vi "2_1_Moving Average system.vi"() -> ()   [LabVIEW 2009]
panel:
  in  "stop":bool
  out "?":dbl[][](graph)=[[1.0, 2.0, 3.0, 2.0, 1.0, 2.0, 7.0, 2.0, 1.0, 3.0, 4.0, -16.0, 2.0, 3.0, -2.0, 5.0, 6.0, 1.0, 20.0, 0.0, 5.0, 2.0, 5.0, -2.0, 1.0, 3.0, -19.0, 2.0, 0.0, 0.0], [1.3333333333333333, 1.5, 1.8333333333333333, 2.8333333333333335, 2.8333333333333335, 2.5, 2.6666666666666665, 3.1666666666666665, 0.16666666666666666, -0.6666666666666666, -0.5, -1.0, -0.6666666666666666, -0.3333333333333333, 2.5, 5.5, 5.0, 6.166666666666667, 5.666666666666667, 5.5, 5.0, 1.8333333333333333, 2.3333333333333335, -1.6666666666666667, -1.6666666666666667, -2.5, -2.1666666666666665, -2.3333333333333335, -2.8333333333333335, 0.3333333333333333]]
  out "Moving Average Output":dbl[](array[numeric])=[1.3333333333333333, 1.5, 1.8333333333333333, 2.8333333333333335, 2.8333333333333335, 2.5, 2.6666666666666665, 3.1666666666666665, 0.16666666666666666, -0.6666666666666666, -0.5, -1.0, -0.6666666666666666, -0.3333333333333333, 2.5, 5.5, 5.0, 6.166666666666667, 5.666666666666667, 5.5, 5.0, 1.8333333333333333, 2.3333333333333335, -1.6666666666666667, -1.6666666666666667, -2.5, -2.1666666666666665, -2.3333333333333335, -2.8333333333333335, 0.3333333333333333]
  in  "M2":dbl=3.0
  in  "M1":dbl=2.0
  in  "Input Signal":dbl[](array[numeric])=[1.0, 2.0, 3.0, 2.0, 1.0, 2.0, 7.0, 2.0, 1.0, 3.0, 4.0, -16.0, 2.0, 3.0, -2.0, 5.0, 6.0, 1.0, 20.0, 0.0, 5.0, 2.0, 5.0, -2.0, 1.0, 3.0, -19.0, 2.0, 0.0, 0.0]
  # "Program Developed by Indranil Sinharoy"
  # "Moving Average System"
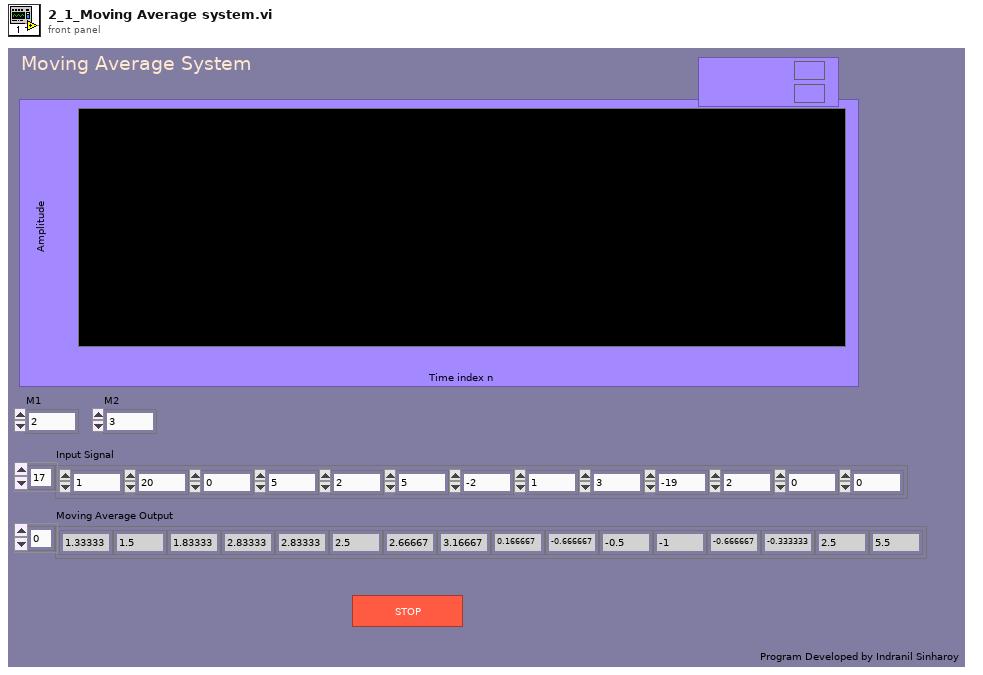
[diagram p1: front panel]
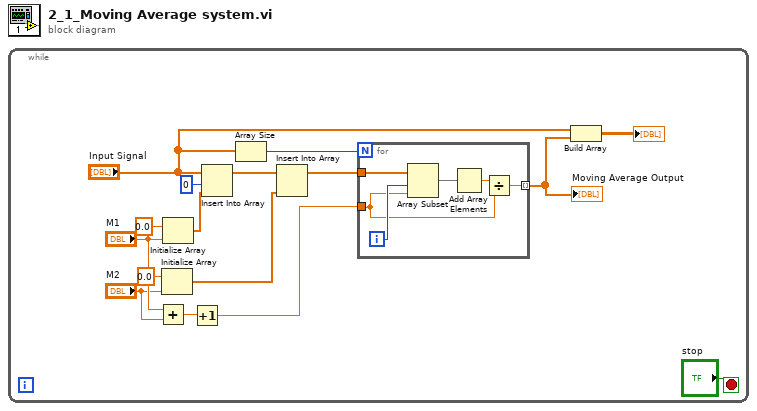
[diagram p0: block diagram]
diagram:
  n1 = while {
    stop <- "stop" stop-if-true
    n2 = Add(x="M1", y="M2") -> (x+y=w7:dbl)
    n3 = Initialize Array(0.0, "M2") -> (w11:dbl[])
    n4 = Initialize Array(0.0, "M1") -> (w15:dbl[])
    n5 = Increment(x=w7) -> (x+1=w5:dbl)
    n6 = Insert Into Array(array="Input Signal", index=0, new element=w15) -> (w13:dbl[])
    n7 = Array Size(array="Input Signal") -> (size(s)=w10:i32)
    n8 = Insert Into Array(array=w13, new element=w11) -> (w6:dbl[])  [unwired: 1 in]
    n9 = for {
      N: w10 -> [_]
      tunnel: w5 -> [w19]
      tunnel: w6 -> [w18]
      tunnel: [w20] -> w4 mode=indexing
      i -> [w22]
      n10 = Array Subset(array=w18, index=w22, length=w19) -> (w17:dbl[])
      n11 = Add Array Elements(numeric array=w17) -> (sum=w21:dbl)
      n12 = Divide(x=w21, y=w19) -> (x/y=w20:dbl)
    }
    "Moving Average Output" <- w4
    n13 = Build Array("Input Signal", w4) -> (→"?":dbl[][])
  }
